vi "bundleField.vi"(8 "error in (no error)":errorcluster, 11 "Field in":refnum<class "Field.lvclass">) -> (0 "error out":errorcluster, 2 "Cluster":T1, 3 "Field out":refnum<class "Field.lvclass">)   [LabVIEW 2018, in "Field.lvclass"]
uses:
  Field.lvclass
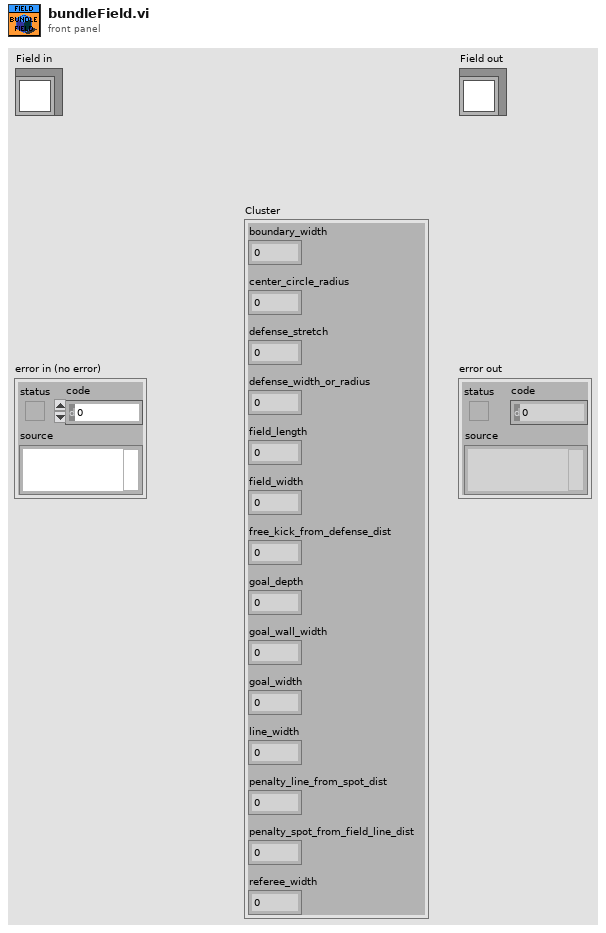
[diagram p1: front panel]
types:
  T1 = cluster{"boundary_width":i32, "center_circle_radius":i32, "defense_stretch":i32, "defense_width_or_radius":i32, "field_length":i32, "field_width":i32, "free_kick_from_defense_dist":i32, "goal_depth":i32, "goal_wall_width":i32, "goal_width":i32, "line_width":i32, "penalty_line_from_spot_dist":i32, "penalty_spot_from_field_line_dist":i32, "referee_width":i32}
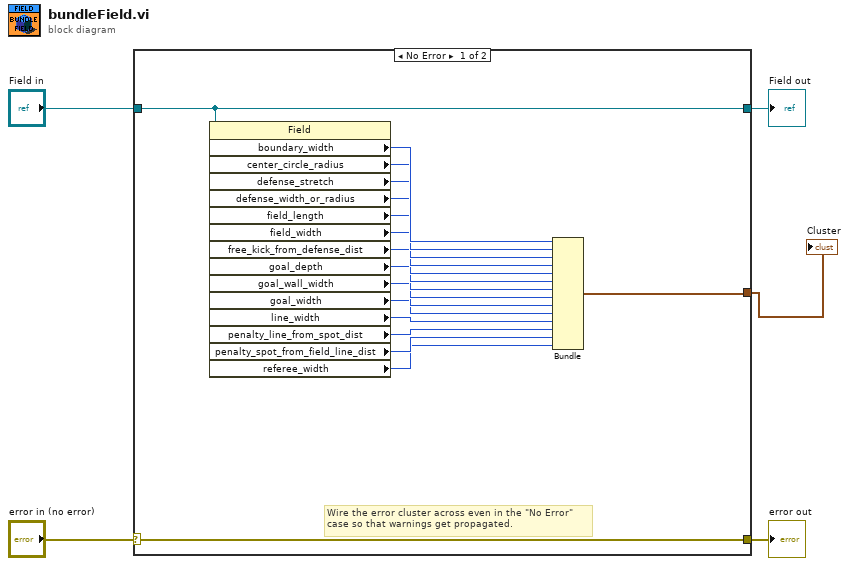
[diagram p0: block diagram]
diagram:
  n1 = case shown="No Error" "error in (no error)" {
    selector: "error in (no error)" -> [w22 w24]
    tunnel: [w22 w24] -> w4
    tunnel: [w21 w23] -> w2
    tunnel: "Field in" -> [w21 w23]
    tunnel: [w6 _] -> w1
    frame No Error {
      # "Wire the error cluster across even in the \"No Error\"\ncase so that warnings get propagated."
      n2 = property class="Field"(reference=w21) -> ("boundary_width"=w20:i32, "center_circle_radius"=w19:i32, "defense_stretch"=w18:i32, "defense_width_or_radius"=w17:i32, "field_length"=w16:i32, "field_width"=w15:i32, "free_kick_from_defense_dist"=w14:i32, "goal_depth"=w13:i32, "goal_wall_width"=w12:i32, "goal_width"=w11:i32, "line_width"=w10:i32, "penalty_line_from_spot_dist"=w9:i32, "penalty_spot_from_field_line_dist"=w8:i32, "referee_width"=w7:i32)  [unwired: 1 in, 2 out]
      n3 = Bundle("boundary_width"=w20, "center_circle_radius"=w19, "defense_stretch"=w18, "defense_width_or_radius"=w17, "field_length"=w16, "field_width"=w15, "free_kick_from_defense_dist"=w14, "goal_depth"=w13, "goal_wall_width"=w12, "goal_width"=w11, "line_width"=w10, "penalty_line_from_spot_dist"=w9, "penalty_spot_from_field_line_dist"=w8, "referee_width"=w7) -> (w6:T1)  [unwired: 1 in]
    }
    frame Error {
    }
  }
  "error out" <- w4
  "Field out" <- w2
  "Cluster" <- w1
